vi "r5y.vi"   [LabVIEW 2019]
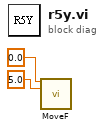
[diagram p0: block diagram]
diagram:
  n1 = call "MoveF.vi"("X"=0.0, "Y"=5.0) -> ()  [unwired: 13 in, 1 out]
